vi "storage.vi"(8 "error in (no error)":errorcluster, 11 "reference in":refnum<class "Project Panels.lvclass">=refnum) -> (0 "error out":errorcluster={"status"=TRUE, "code"=1556, "source"="In Place Element Structure in Project Panels.lvclass:items.vi"}, 2 "saved?":bool, 3 "reference out":refnum<class "Project Panels.lvclass">)   [LabVIEW 2015, in "Project Panels.lvclass"]
uses:
  Project Panels.lvclass
  SYS/Items Controller_llb/storageSheets.ctl
  stateItem.ctl
  <vilib>/Utility/miscctls.llb/LVRowAndColumnUnsignedTypeDef.ctl
  <vilib>/Utility/miscctls.llb/LVRowAndColumnTypeDef.ctl
  SYS/Items Controller_llb/Items Controller.lvclass
  SYS/File Controller_llb/File Controller.lvclass
panel:
  out "title":string="Cosmed Asia Pacific - Storage"
  in  "tables":enum32{"Check IN", "Check OUT", "Storage"}(tab)
  in  "checkIN":string[][](table)
  in  "checkOUT":string[][](table)
  in  "Storage":string[][](table)
  in  "uploadFile":bool
  in  "Add Check OUT":bool
  in  "Add Check IN":bool
  out "Number of Items:":i32
  out "index":i32
  in  "back":bool
  in  "next":bool
  out "storageSheets":T1
  in  "Search Item":bool
  in  "Save":bool
  out "Item Selected (S/N or P/N):":string
  out "statuBar":string="Stoped for an Error"
  in  "Stop Button":bool
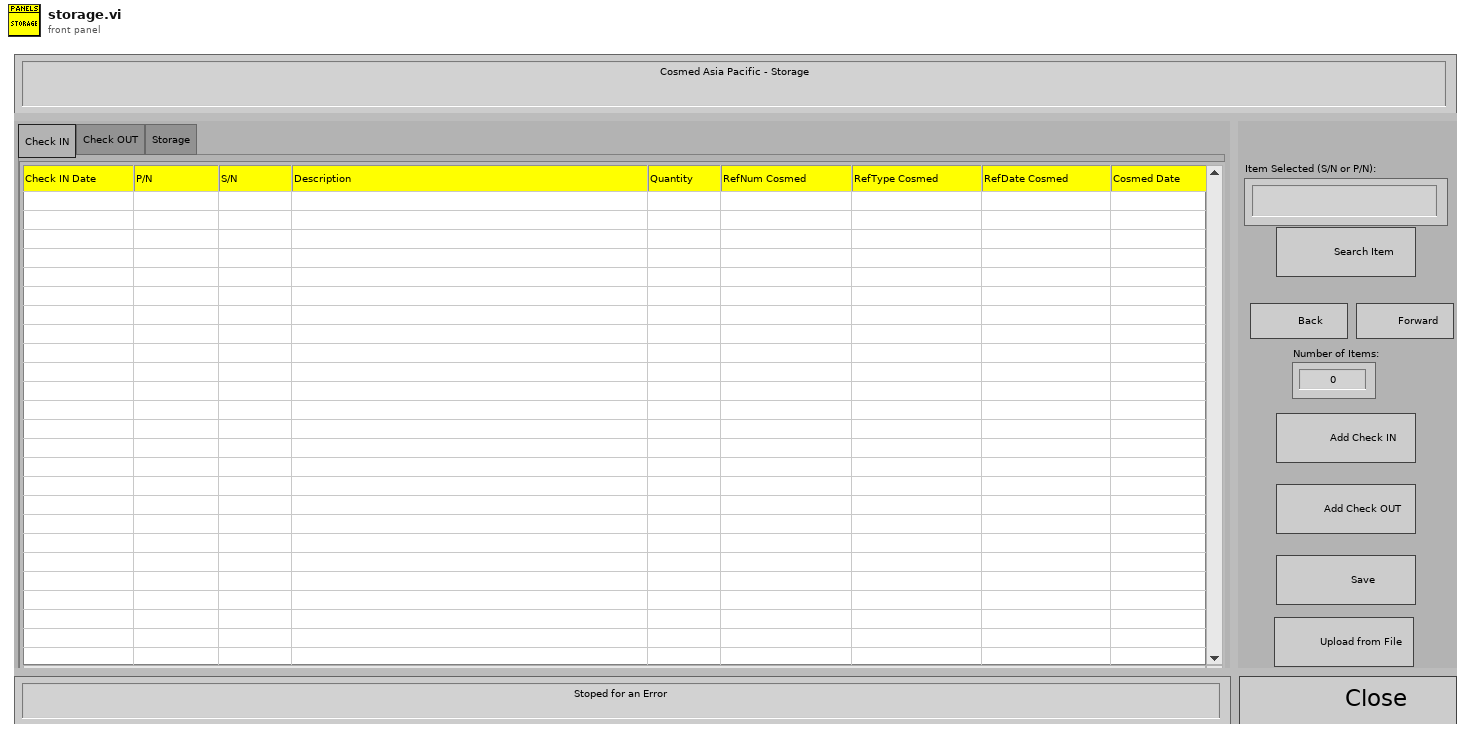
[diagram p1: front panel]
types:
  T1 = typedef "Items Controller.lvclass/storageSheets.ctl" = enum16{"check-in", "check-out", "storage"}
  T2 = typedef "Project Panels.lvclass/stateItem.ctl" = enum16{"initiate", "waitEvent", "save", "search", "UploadFile", "nextItems", "stop"}
  T3 = typedef "LVRowAndColumnUnsignedTypeDef.ctl" = cluster{"Row":u32, "Column":u32}
  T4 = enum8{"Enabled", "Disabled", "Disabled and Grayed Out"}
  T5 = cluster{"checkIN":string[][], "checkOUT":string[][], "storage":string[][]}
  T6 = typedef "LVRowAndColumnTypeDef.ctl" = cluster{"Row":i32, "Column":i32}
  T7 = typedef "Project Panels.lvclass/ObjectAttributesRef.ctl" = refnum<data-value>
  T8 = typedef "Project Panels.lvclass/ObjectAttributes.ctl" = cluster{"MyAttribute":dbl, "device_controller_ref":refnum<class "Devices Controller.lvclass">, "file_controller_ref":refnum<class "File Controller.lvclass">, "item_controller_ref":refnum<class "Items Controller.lvclass">, "item_tables":cluster{"checkIN":string[][], "checkOUT":string[][], "storage":string[][]}, "quickbook_table":cluster{"notes":string[][]}, "notification_controller_ref":refnum<class "Notification Controller.lvclass">, "partstracking_controller_ref":refnum<class "PartsTracking Controller.lvclass">, "product_tables":cluster{"k4b2":string[][], "fitmate":string[][], "RMR":string[][], "CPET":string[][], "BP":string[][], "PP":string[][], "k5":string[][], "bb-pft":string[][]}, "rowsColour":u32[], "low_resolution?":bool, "run_python?":bool}
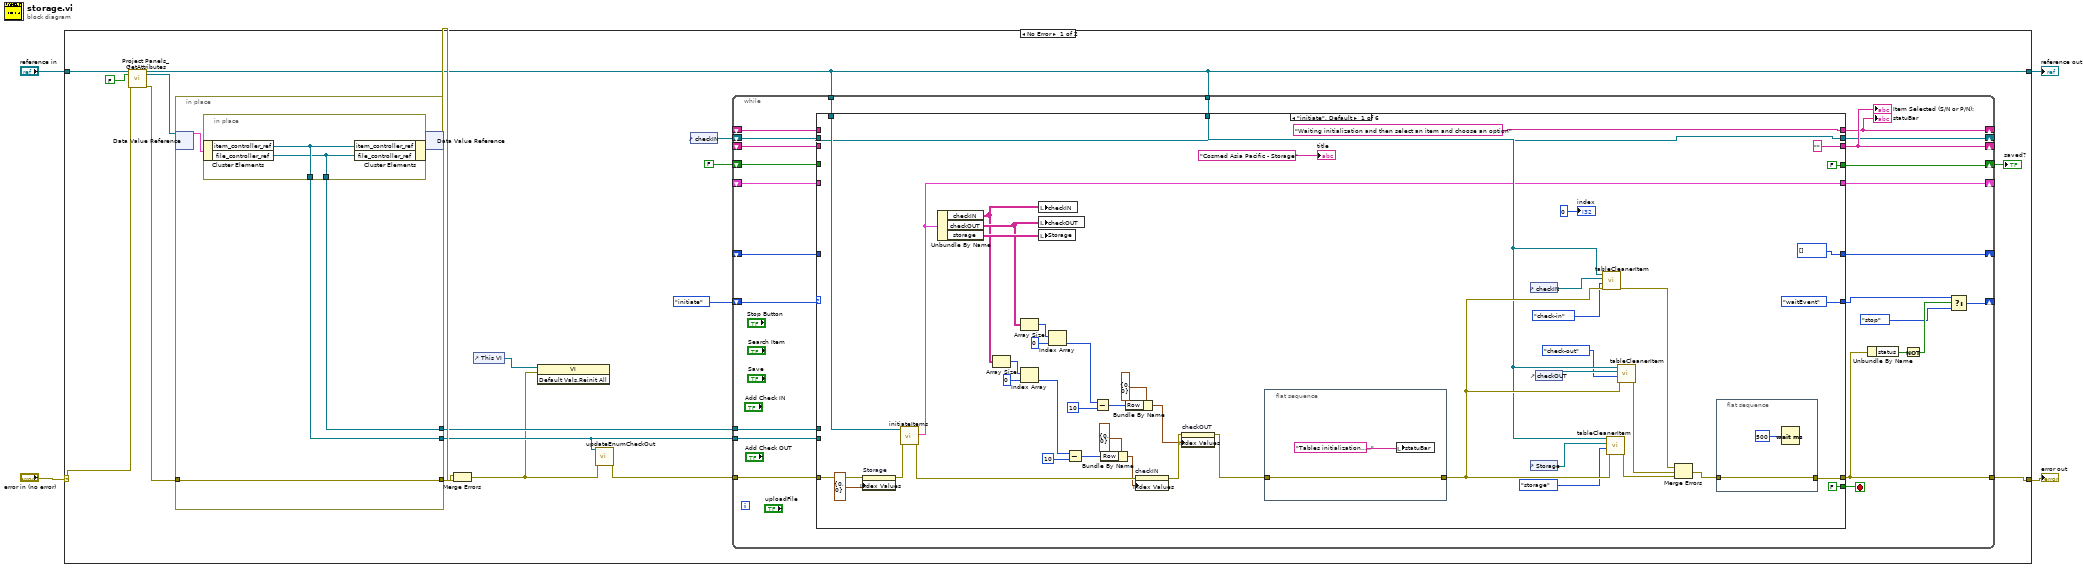
[diagram p0: block diagram]
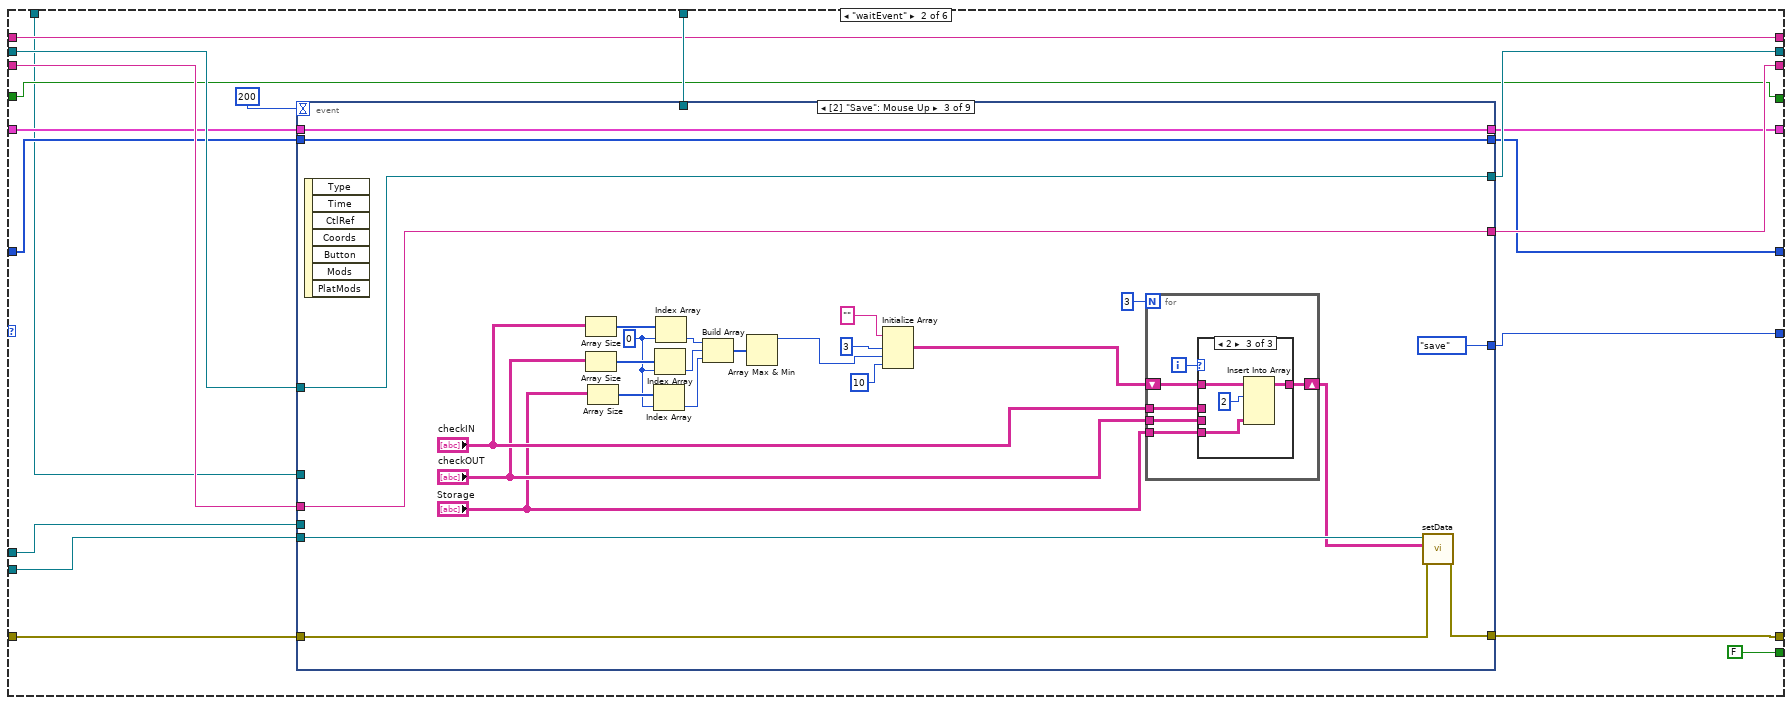
[diagram p2: hidden frame]
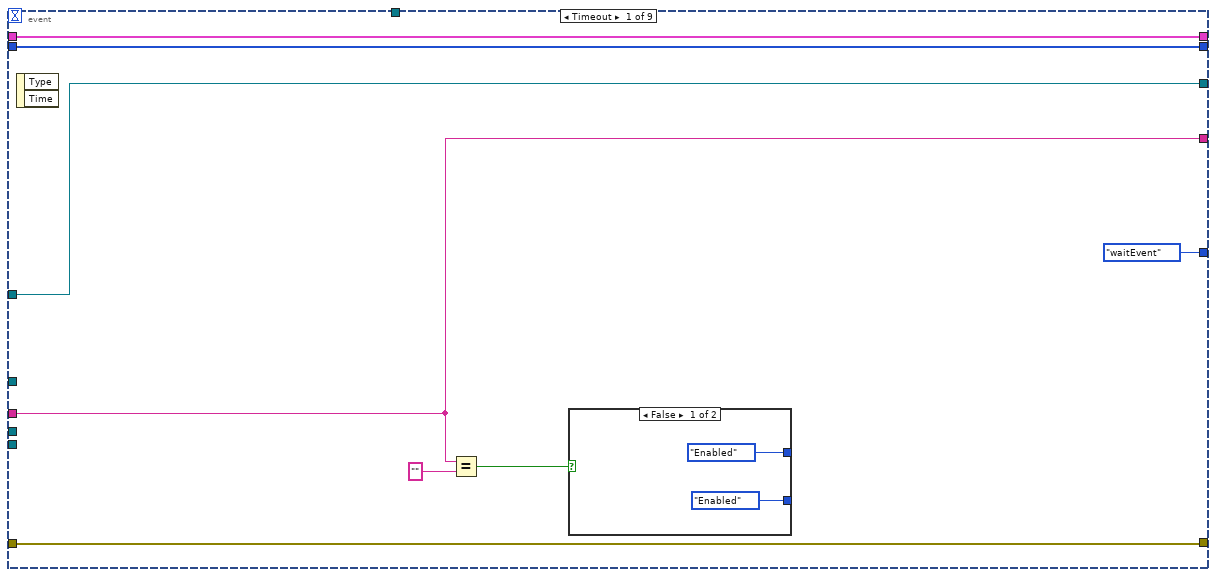
[diagram p3: hidden frame]
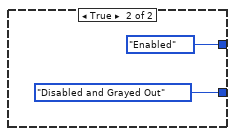
[diagram p4: hidden frame]
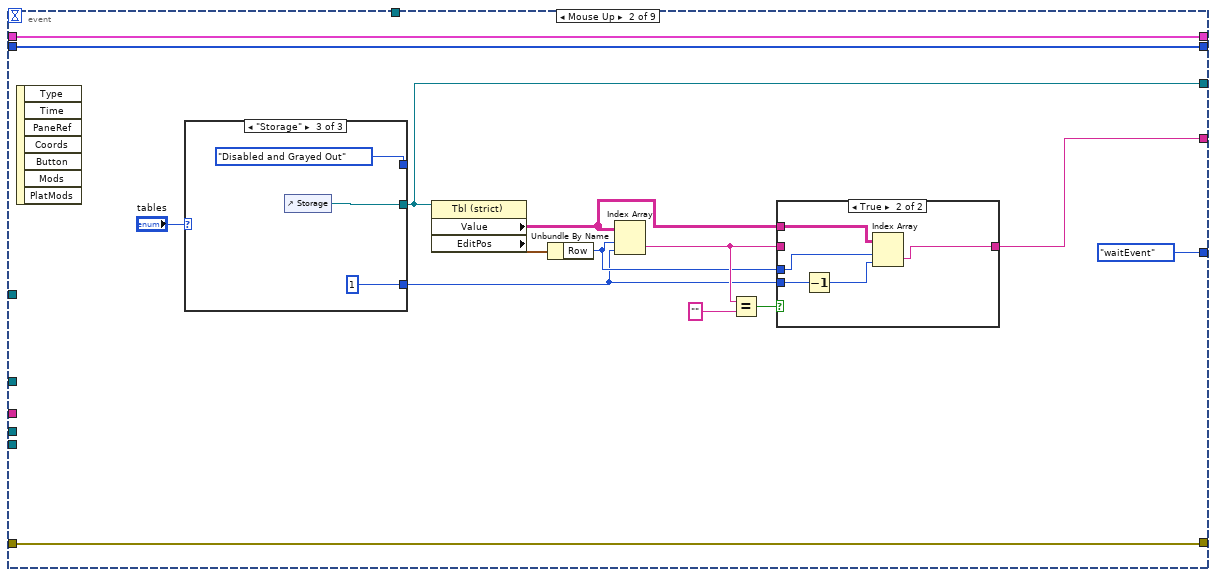
[diagram p5: hidden frame]
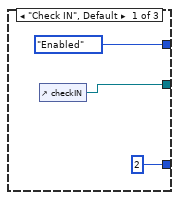
[diagram p7: hidden frame]
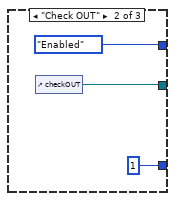
[diagram p8: hidden frame]
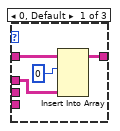
[diagram p9: hidden frame]
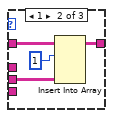
[diagram p10: hidden frame]
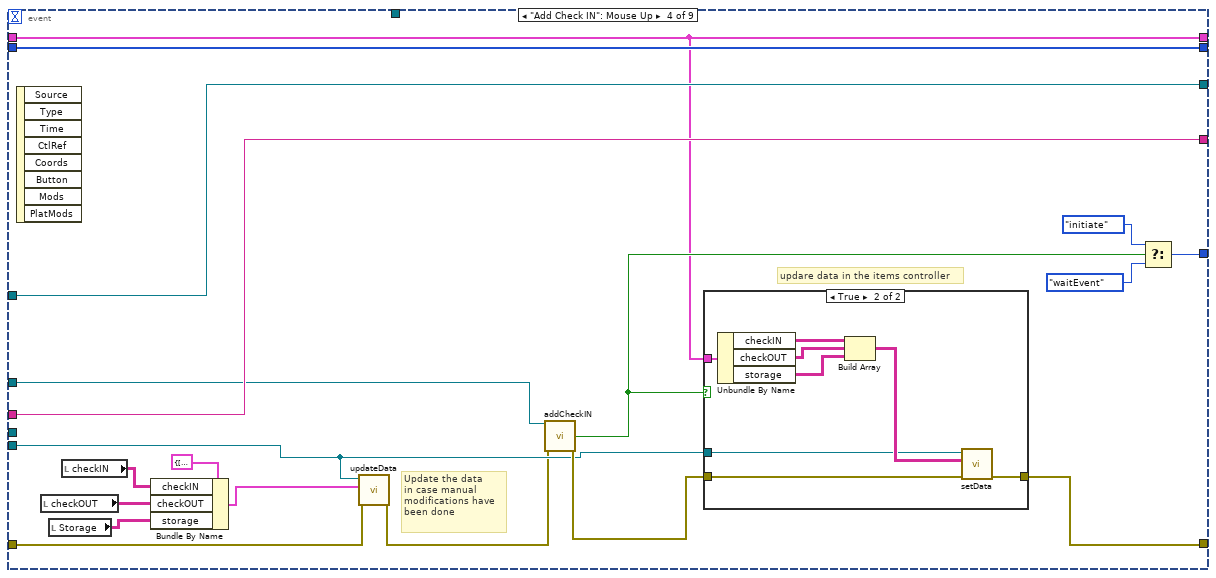
[diagram p11: hidden frame]
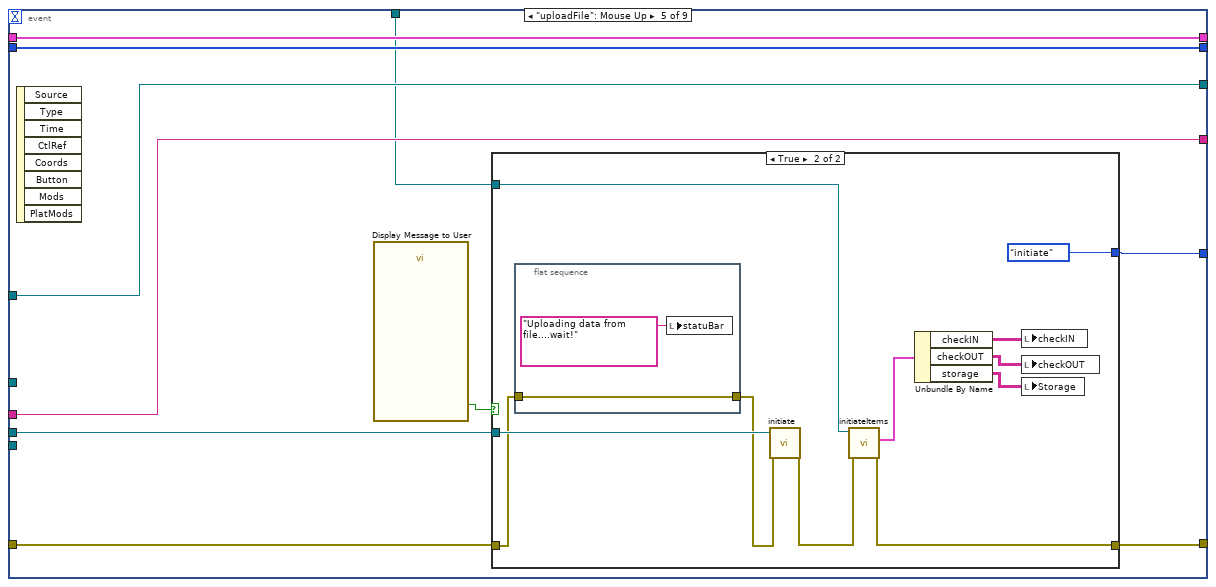
[diagram p13: hidden frame]
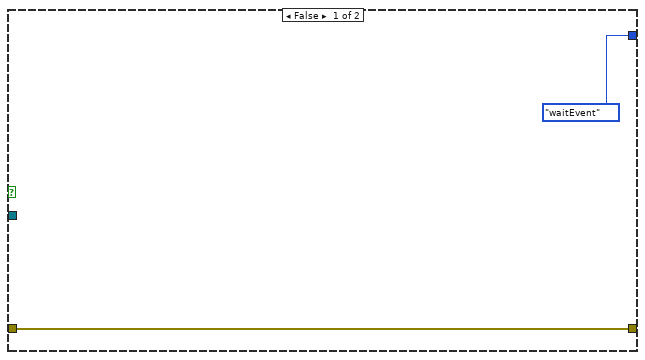
[diagram p14: hidden frame]
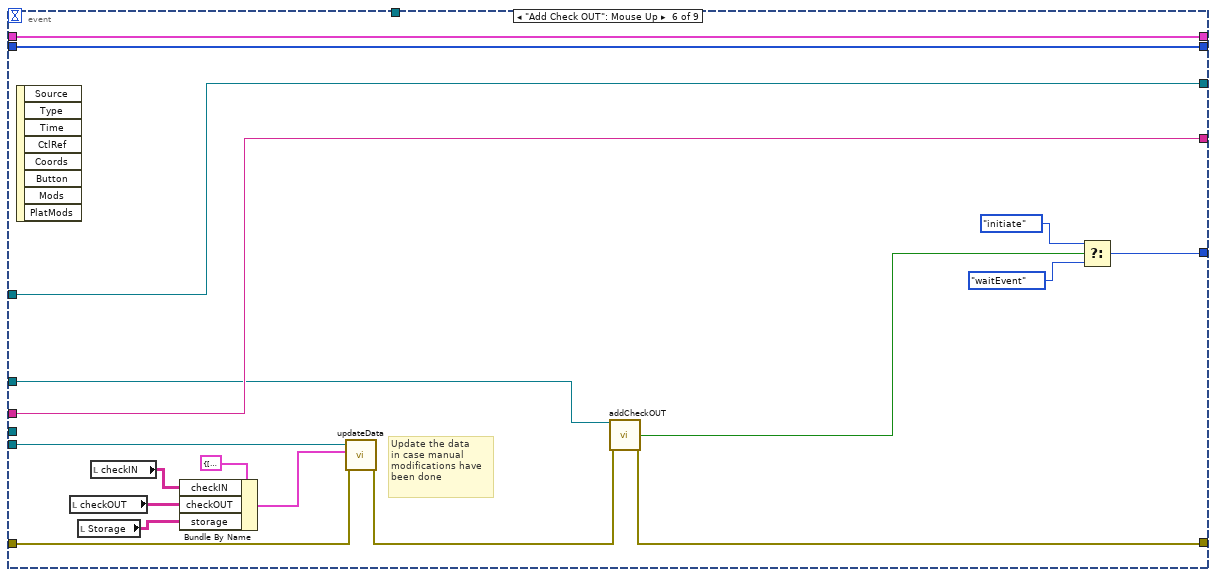
[diagram p15: hidden frame]
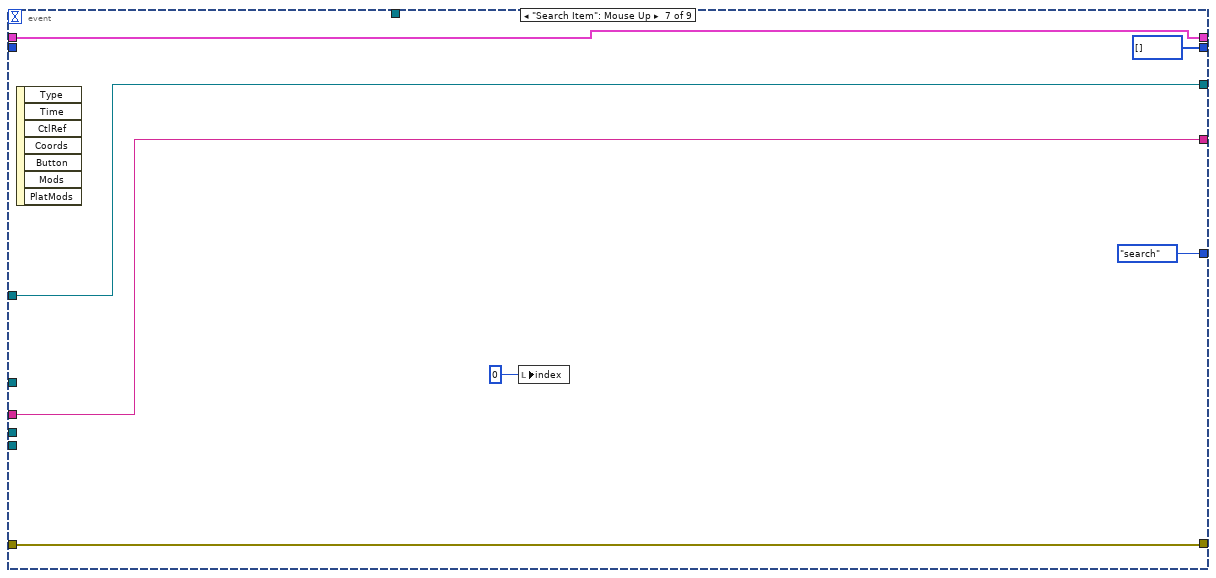
[diagram p16: hidden frame]
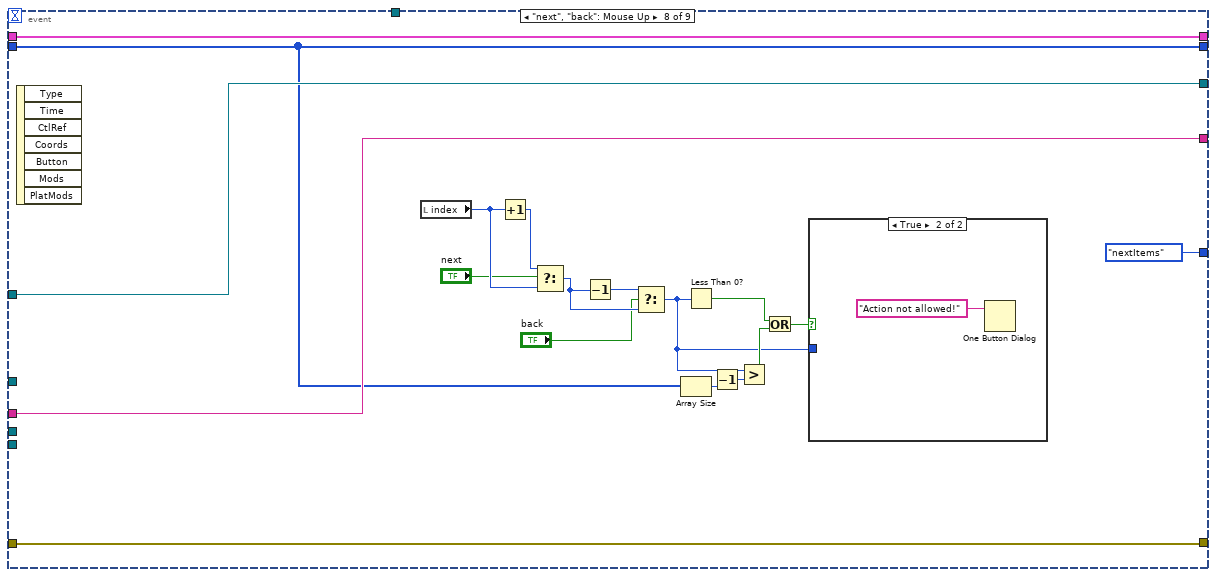
[diagram p17: hidden frame]
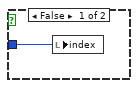
[diagram p18: hidden frame]
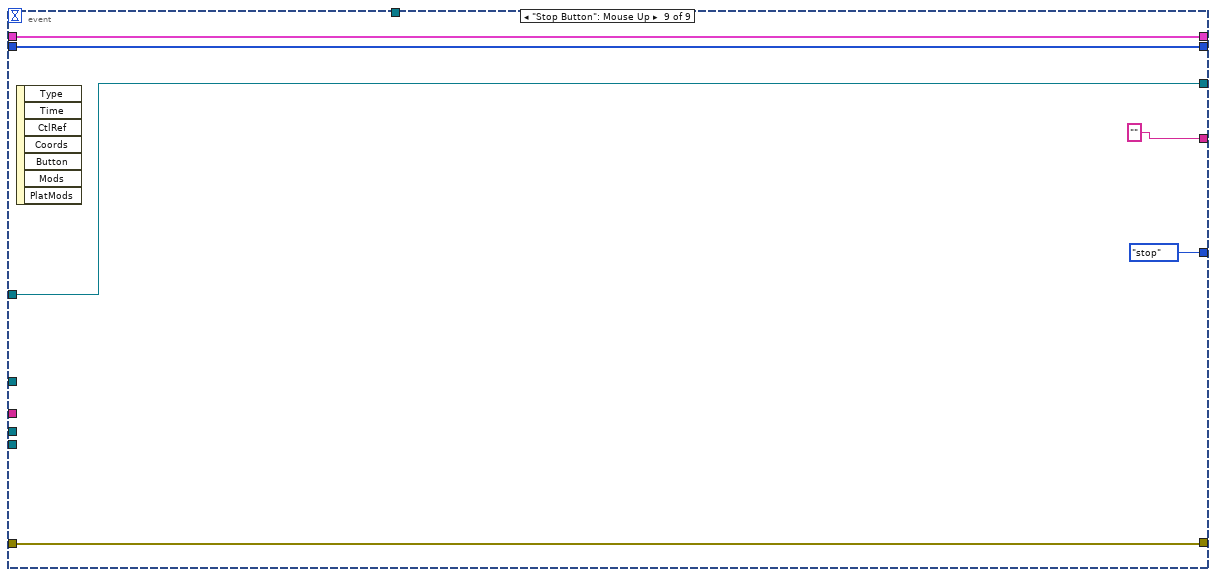
[diagram p19: hidden frame]
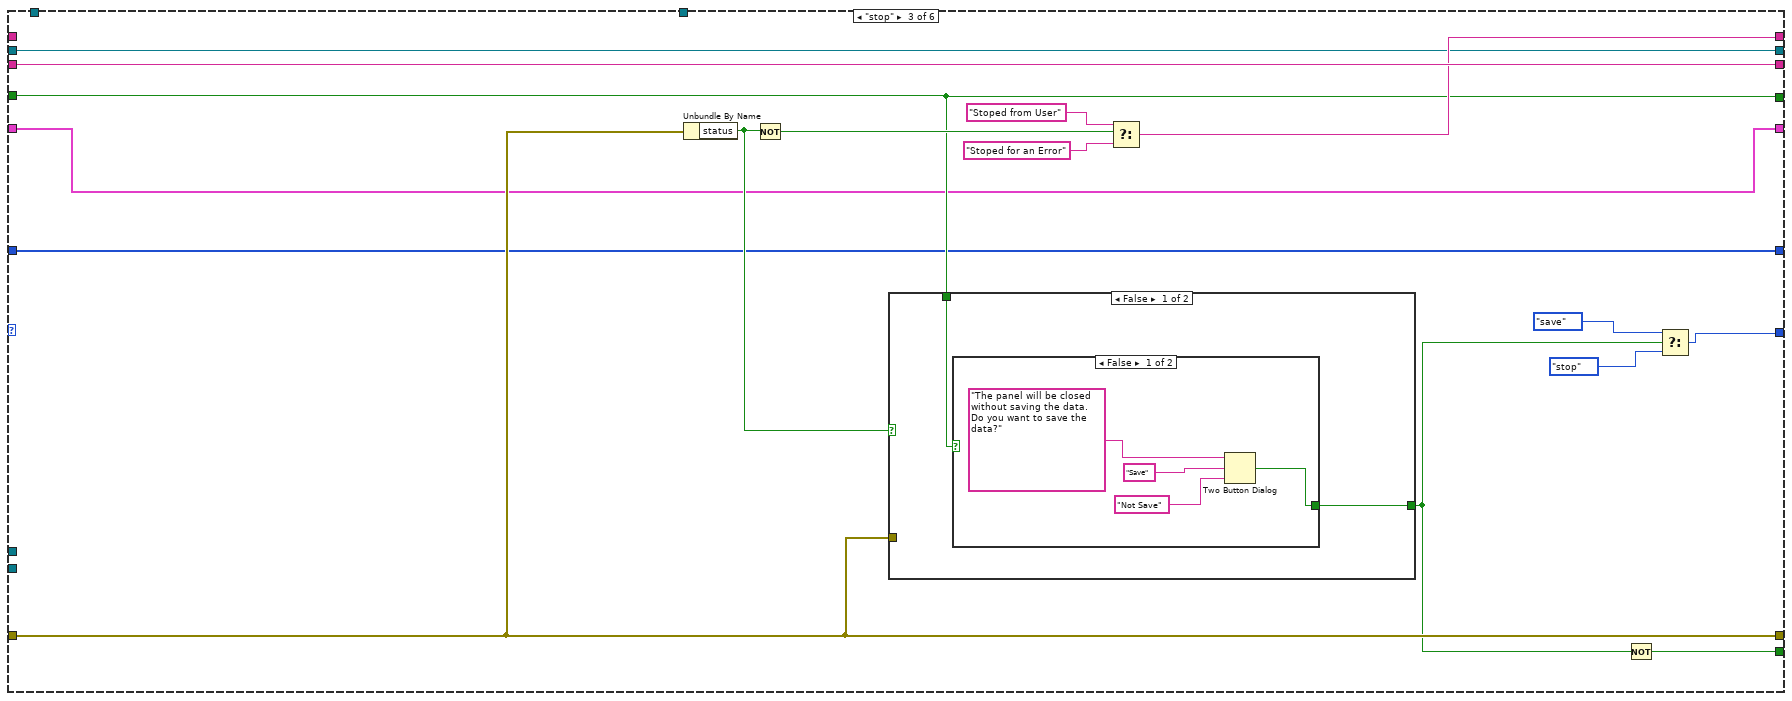
[diagram p20: hidden frame]
diagram:
  n1 = case shown="No Error" "error in (no error)" {
    selector: "error in (no error)" -> [w18 w401]
    tunnel: [w15 w401] -> w3
    tunnel: [w13 w400] -> w1
    tunnel: "reference in" -> [w20 w400]
    frame No Error {
      n2 = call "Project Panels_GetAttributes.vi"("reference in"=w20, "return data? (T)"=FALSE, "error in (no error)"=w18) -> ("reference out"=w13:refnum<class "Project Panels.lvclass">, "attributes ref"=w16:T7, "error out"=w17:errorcluster)  [unwired: 13 in, 1 out]
      n3 = in-place {
        in-place-border: w17 -> [w395]
        in-place-border: [w395] -> w21
        in-place-border: [w394] -> w7
        in-place-border: [w393] -> w8
        n4 = in-place-dvr #1(w16) -> (w396:T8)  [unwired: 1 out]
        n5 = in-place {
          in-place-border: [w399] -> w394
          in-place-border: [w398] -> w393
          n6 = in-place-cluster #2(w396) -> ("item_controller_ref"=w399:refnum<class "Items Controller.lvclass">, "file_controller_ref"=w398:refnum<class "File Controller.lvclass">)
          n7 = in-place-cluster #2("item_controller_ref"=w399, "file_controller_ref"=w398) -> (w397:T8)
        }
        n8 = in-place-dvr #1(w397) -> (w22:errorcluster)  [unwired: 1 out]
      }
      n9 = Merge Errors(w21, w22) -> (w6:errorcluster)
      n10 = control-ref of="This VI"() -> (w11:refnum<vi>)
      n11 = invoke class="VI" method="Default Vals.Reinit All"(reference=w11, error in=w6) -> ()  [unwired: 1 in, 3 out]
      n12 = call "updateEnumCheckOut.vi"("reference in"=w7, "error in (no error)"=w6) -> ("error out"=w5:errorcluster)  [unwired: 16 in, 1 out]
      n13 = control-ref of="checkIN"() -> (w12:refnum<vi>)
      n14 = while {
        tunnel: w13 -> [w47]
        tunnel: w5 -> [w46]
        tunnel: [w44] -> w15
        shift-right: [w41] -> _
        shift-left: stateItem."initiate" ("state") -> [w45]
        shift-right: [w38] -> _
        shift-left: _ -> [w37]
        shift-right: [w36] -> _
        shift-left: w12 -> [w35]
        tunnel: w13 -> [w34]
        tunnel: w7 -> [w32]
        shift-right: [w30] -> w9
        shift-left: FALSE -> [w31]
        shift-right: [w29] -> _
        shift-left: _ -> [w28]
        shift-right: [w27] -> _
        shift-left: _ -> [w26]
        shift-right: [w25] -> _
        shift-left: _ -> [w24]
        tunnel: w8 -> [w23]
        stop <- w39 stop-if-true
        n15 = case shown="\"initiate\", Default" w45 {
          tunnel: w47 -> [w82 w107 _ _ _ _]
          tunnel: w46 -> [w75 w116 w317 w335 w367 w383]
          tunnel: [w85 w110 w317 w346 w367 w379] -> w44
          tunnel: [stateItem."waitEvent" ("state") w109 w312 w341 stateItem."waitEvent" ("state") stateItem."waitEvent" ("state")] -> w42
          tunnel: [FALSE FALSE w310 FALSE FALSE FALSE] -> w39
          tunnel: ["Waiting initialization and then select an item and choose an option" ("title") w105 w319 "Search Item option selected..." ("title") "Click on the arrows to select other items" ("title") w378] -> w29
          tunnel: ["" w112 w322 w347 w364 w385] -> w38
          tunnel: w37 -> [_ w114 w322 w347 w364 w385]
          tunnel: [w79 w111 w318 w348 w358 w386] -> w36
          tunnel: w35 -> [w79 w113 w318 w348 w358 w386]
          tunnel: w34 -> [w81 w100 _ w337 _ _]
          tunnel: w32 -> [_ w108 _ _ _ w384]
          tunnel: w31 -> [_ w106 w309 w345 w365 _]
          tunnel: [FALSE w106 w309 w345 w365 TRUE] -> w30
          tunnel: w28 -> [_ w105 _ _ _ _]
          tunnel: [i32[] [] ("indexElements") w103 w308 w339 w359 w380] -> w27
          tunnel: w26 -> [_ w104 w308 _ w359 w380]
          tunnel: [w48 w101 w307 w336 w351 w377] -> w25
          tunnel: w24 -> [_ w102 w307 w336 w351 w377]
          tunnel: w23 -> [_ w99 _ _ _ _]
          frame "initiate", Default {
            n16 = property on="Storage" class="Tbl (strict)"(error in=w75, "Index Values"=T3 {"Row"=0, "Column"=0}) -> (error out=w74:errorcluster)  [unwired: 1 in, 1 out]
            n17 = call "initiateItems.vi"("error in (no error)"=w74, "reference in"=w81) -> ("error out"=w66:errorcluster, "table"=w48:T5)  [unwired: 7 in, 1 out]
            n18 = Unbundle By Name(w48) -> ("checkIN"=w49:string[][], "checkOUT"=w68:string[][], "storage"=w73:string[][])
            n19 = Array Size(array=w49) -> (size(s)=w55:i32[])
            n20 = Array Size(array=w68) -> (size(s)=w62:i32[])
            n21 = Index Array(array=w55, index=0) -> (element=w52:i32)
            n22 = local write "checkIN"(w49) -> ()
            n23 = local write "checkOUT"(w68) -> ()
            n24 = local write "Storage"(w73) -> ()
            n25 = Index Array(array=w62, index=0) -> (element=w59:i32)
            n26 = Subtract(x=w52, y=10) -> (x-y=w53:i32)
            n27 = Subtract(x=w59, y=10) -> (x-y=w60:i32)
            n28 = Bundle By Name(cluster=T3 {"Row"=0, "Column"=0} ("Index Values"), "Row"=w53) -> (w50:T3)
            n29 = Bundle By Name(cluster=T3 {"Row"=0, "Column"=0} ("Index Values"), "Row"=w60) -> (w57:T3)
            n30 = property on="checkIN" class="Tbl (strict)"(error in=w66, "Index Values"=w50) -> (error out=w65:errorcluster)  [unwired: 1 in, 1 out]
            n31 = property on="checkOUT" class="Tbl (strict)"(error in=w65, "Index Values"=w57) -> (error out=w67:errorcluster)  [unwired: 1 in, 1 out]
            n32 = flat-sequence {
              tunnel: w67 -> [w96]
              tunnel: [w96] -> w84
              frame #0 {
                n33 = local write "statuBar"("Tables initialization....." ("title")) -> ()
              }
            }
            n34 = control-ref of="checkIN"() -> (w92:refnum<vi>)
            n35 = control-ref of="Storage"() -> (w94:refnum<vi>)
            n36 = control-ref of="checkOUT"() -> (w93:refnum<vi>)
            n37 = call "tableCleanerItem.vi"("error in (no error)"=w84, "storageSheets"=storageSheets."check-in", "Table in"=w92, "reference in"=w82) -> ("error out"=w91:errorcluster)  [unwired: 6 in, 1 out]
            n38 = call "tableCleanerItem.vi"("error in (no error)"=w84, "storageSheets"=storageSheets."storage", "Table in"=w94, "reference in"=w82) -> ("error out"=w89:errorcluster)  [unwired: 6 in, 1 out]
            n39 = call "tableCleanerItem.vi"("error in (no error)"=w84, "storageSheets"=storageSheets."check-out", "Table in"=w93, "reference in"=w82) -> ("error out"=w90:errorcluster)  [unwired: 6 in, 1 out]
            n40 = Merge Errors(w91, w90, w89) -> (w80:errorcluster)
            n41 = flat-sequence {
              tunnel: w80 -> [w98]
              tunnel: [w98] -> w85
              frame #0 {
                n42 = Wait (ms)(milliseconds to wait=u32 500) -> ()  [unwired: 1 out]
              }
            }
            "title" <- "Cosmed Asia Pacific - Storage" ("title")
            "index" <- 0 ("index")
          }
          frame "waitEvent" {
            n43 = event shown="[2] \"Save\": Mouse Up" {
              selector: _ -> [_ _ _ _ _ _ _ _ _]
              dyn-events: _ -> [_ _ _ _ _ _ _ _ _]
              timeout: 200 -> [_ _ _ _ _ _ _ _ _]
              tunnel: w116 -> [w125 w143 w180 w209 w236 w264 w277 w298 w306]
              tunnel: [w125 w143 w179 w212 w235 w269 w277 w298 w306] -> w110
              tunnel: w114 -> [w121 _ w183 w221 w237 w273 w279 w291 _]
              tunnel: w113 -> [w122 _ w184 w220 w238 w272 w280 w292 w304]
              tunnel: [w121 w136 w183 w221 w237 w273 w279 w291 ""] -> w112
              tunnel: [w122 w140 w184 w220 w238 w272 w280 w292 w304] -> w111
              tunnel: [stateItem."waitEvent" ("state") stateItem."waitEvent" ("state") stateItem."save" ("state") w216 w233 w267 stateItem."search" ("state") stateItem."nextItems" ("state") stateItem."stop" ("state")] -> w109
              tunnel: w108 -> [_ _ w178 w211 _ w262 _ _ _]
              tunnel: w107 -> [_ _ _ _ w231 _ _ _ _]
              tunnel: w104 -> [w119 w131 w176 w219 w239 w271 _ w290 w302]
              tunnel: [w119 w131 w176 w219 w239 w271 i32[] [] ("indexElements") w290 w302] -> w103
              tunnel: w102 -> [w118 w130 w175 w210 w240 w261 w274 w281 w301]
              tunnel: [w118 w130 w175 w210 w240 w261 w274 w281 w301] -> w101
              tunnel: w100 -> [_ _ _ w218 _ w270 _ _ _]
              tunnel: w99 -> [_ _ _ _ w232 _ _ _ _]
              event Timeout {
                n44 = event-data() -> ()  [unwired: 1 in, 2 out]
                n45 = Equal?(x=w121, y="") -> (x = y?=w124:bool)
                n46 = case shown="False" w124 {
                  tunnel: [T4."Enabled" ("Disabled") T4."Disabled and Grayed Out" ("Disabled")] -> _
                  tunnel: [T4."Enabled" ("Disabled") T4."Enabled" ("Disabled")] -> _
                  frame False {
                  }
                  frame True {
                  }
                }
              }
              event Mouse Up {
                n47 = event-data() -> ()  [unwired: 1 in, 7 out]
                n48 = case shown="\"Storage\"" "tables" {
                  tunnel: [w152 w155 w158] -> w140
                  tunnel: [T4."Enabled" ("Disabled") T4."Enabled" ("Disabled") T4."Disabled and Grayed Out" ("Disabled")] -> _
                  tunnel: [2 ("disabled index (col)") 1 ("disabled index (col)") 1 ("disabled index (col)")] -> w133
                  frame "Check IN", Default {
                    n49 = control-ref of="checkIN"() -> (w152:refnum<vi>)
                  }
                  frame "Check OUT" {
                    n50 = control-ref of="checkOUT"() -> (w155:refnum<vi>)
                  }
                  frame "Storage" {
                    n51 = control-ref of="Storage"() -> (w158:refnum<vi>)
                  }
                }
                n52 = property on="Property Node" class="Tbl (strict)"(reference=w140) -> ("Value"=w135:string[][], "EditPos"=w142:T6)  [unwired: 1 in, 2 out]
                n53 = Unbundle By Name(w142) -> ("Row"=w134:i32)
                n54 = Index Array(array=w135, index (row)=w134, index (col)=w133) -> (element=w137:string)
                n55 = Equal?(x=w137, y="") -> (x = y?=w138:bool)
                n56 = case shown="True" w138 {
                  tunnel: w137 -> [w144 _]
                  tunnel: [w144 w145] -> w136
                  tunnel: w135 -> [_ w149]
                  tunnel: w134 -> [_ w148]
                  tunnel: w133 -> [_ w147]
                  frame False {
                  }
                  frame True {
                    n57 = Decrement(x=w147) -> (x-1=w146:i32)
                    n58 = Index Array(array=w149, index (row)=w148, index (col)=w146) -> (element=w145:string)
                  }
                }
              }
              event "Save": Mouse Up {
                w168 = 0 ("index")
                n59 = event-data() -> ()  [unwired: 1 in, 7 out]
                n60 = Array Size(array="checkIN") -> (size(s)=w171:i32[])
                n61 = Array Size(array="checkOUT") -> (size(s)=w170:i32[])
                n62 = Array Size(array="Storage") -> (size(s)=w169:i32[])
                n63 = Index Array(array=w169, index=w168) -> (element=w165:i32)
                n64 = Index Array(array=w170, index=w168) -> (element=w166:i32)
                n65 = Index Array(array=w171, index=w168) -> (element=w167:i32)
                n66 = Build Array(w167, w166, w165) -> (w164:i32[])
                n67 = Array Max & Min(array=w164) -> (max value=w161:i32)  [unwired: 3 out]
                n68 = Initialize Array("", 3 ("dimension size"), w161, 10 ("dimension size")) -> (w159:string[][][])
                n69 = for {
                  N: 3 -> [_]
                  shift-right: [w187] -> w177
                  shift-left: w159 -> [w189]
                  tunnel: "checkIN" -> [w188]
                  tunnel: "checkOUT" -> [w186]
                  tunnel: "Storage" -> [w185]
                  i -> [w190]
                  n70 = case shown="2" w190 {
                    tunnel: w189 -> [w194 w198 w202]
                    tunnel: w188 -> [w191 _ _]
                    tunnel: [w193 w197 w201] -> w187
                    tunnel: w186 -> [_ w195 _]
                    tunnel: w185 -> [_ _ w199]
                    frame 0, Default {
                      n71 = Insert Into Array(array=w194, index (dim 0)=0 ("index (page)"), new element=w191) -> (w193:string[][][])  [unwired: 2 in]
                    }
                    frame 1 {
                      n72 = Insert Into Array(array=w198, index (dim 0)=1 ("disabled index (page)"), new element=w195) -> (w197:string[][][])  [unwired: 2 in]
                    }
                    frame 2 {
                      n73 = Insert Into Array(array=w202, index (dim 0)=2 ("disabled index (page)"), new element=w199) -> (w201:string[][][])  [unwired: 2 in]
                    }
                  }
                }
                n74 = call "setData.vi"("error in (no error)"=w180, "data"=w177, "reference in"=w178) -> ("error out"=w179:errorcluster)  [unwired: 7 in, 1 out]
              }
              event "Add Check IN": Mouse Up {
                # "Update the data\nin case manual\nmodifications have\nbeen done"
                # "updare data in the items controller"
                n75 = event-data() -> ()  [unwired: 1 in, 8 out]
                n76 = local read "checkOUT"() -> (w205:string[][])
                n77 = local read "Storage"() -> (w204:string[][])
                n78 = local read "checkIN"() -> (w206:string[][])
                n79 = Bundle By Name(cluster=T5 {"checkIN"=[], "checkOUT"=[], "storage"=[]} ("table"), "checkIN"=w206, "checkOUT"=w205, "storage"=w204) -> (w203:T5)
                n80 = call "updateData.vi"("error in (no error)"=w209, "table"=w203, "reference in"=w211) -> ("error out"=w208:errorcluster)  [unwired: 7 in, 1 out]
                n81 = call "addCheckIN.vi"("reference in"=w218, "error in (no error)"=w208) -> ("saved?"=w214:bool, "error out"=w213:errorcluster)  [unwired: 11 in, 1 out]
                n82 = case shown="True" w214 {
                  tunnel: w210 -> [_ w226]
                  tunnel: w213 -> [w222 w225]
                  tunnel: [w222 w224] -> w212
                  tunnel: w211 -> [_ w223]
                  frame False {
                  }
                  frame True {
                    n83 = Unbundle By Name(w226) -> ("checkIN"=w230:string[][], "checkOUT"=w229:string[][], "storage"=w228:string[][])
                    n84 = Build Array(w230, w229, w228) -> (w227:string[][][])
                    n85 = call "setData.vi"("error in (no error)"=w225, "data"=w227, "reference in"=w223) -> ("error out"=w224:errorcluster)  [unwired: 7 in, 1 out]
                  }
                }
                n86 = Select(t=stateItem."initiate" ("state"), s=w214, f=stateItem."waitEvent") -> (s? t:f=w216:T2)
              }
              event "uploadFile": Mouse Up {
                n87 = event-data() -> ()  [unwired: 1 in, 8 out]
                n88 = call "Display Message to User"() -> ("Yes"=w234:bool)  [unwired: 10 in, 1 out]
                n89 = case shown="True" w234 {
                  tunnel: w236 -> [w242 w244]
                  tunnel: [w242 w248] -> w235
                  tunnel: [stateItem."waitEvent" ("state") stateItem."initiate" ("state")] -> w233
                  tunnel: w232 -> [_ w252]
                  tunnel: w231 -> [_ w250]
                  frame False {
                  }
                  frame True {
                    n90 = flat-sequence {
                      tunnel: w244 -> [w255]
                      tunnel: [w255] -> w243
                      frame #0 {
                        n91 = local write "statuBar"("Uploading data from file....wait!" ("statuBar")) -> ()
                      }
                    }
                    n92 = call "initiate.vi"("reference in"=w252, "error in (no error)"=w243) -> ("error out"=w249:errorcluster)  [unwired: 16 in, 1 out]
                    n93 = call "initiateItems.vi"("error in (no error)"=w249, "reference in"=w250) -> ("error out"=w248:errorcluster, "table"=w251:T5)  [unwired: 7 in, 1 out]
                    n94 = Unbundle By Name(w251) -> ("checkIN"=w247:string[][], "checkOUT"=w246:string[][], "storage"=w245:string[][])
                    n95 = local write "checkIN"(w247) -> ()
                    n96 = local write "checkOUT"(w246) -> ()
                    n97 = local write "Storage"(w245) -> ()
                  }
                }
              }
              event "Add Check OUT": Mouse Up {
                # "Update the data\nin case manual\nmodifications have\nbeen done"
                n98 = event-data() -> ()  [unwired: 1 in, 8 out]
                n99 = local read "checkOUT"() -> (w258:string[][])
                n100 = local read "Storage"() -> (w257:string[][])
                n101 = local read "checkIN"() -> (w259:string[][])
                n102 = Bundle By Name(cluster=T5 {"checkIN"=[], "checkOUT"=[], "storage"=[]} ("table"), "checkIN"=w259, "checkOUT"=w258, "storage"=w257) -> (w256:T5)
                n103 = call "updateData.vi"("error in (no error)"=w264, "table"=w256, "reference in"=w262) -> ("error out"=w263:errorcluster)  [unwired: 7 in, 1 out]
                n104 = call "addCheckOUT.vi"("reference in"=w270, "error in (no error)"=w263) -> ("saved?"=w266:bool, "error out"=w269:errorcluster)  [unwired: 11 in, 1 out]
                n105 = Select(t=stateItem."initiate" ("state"), s=w266, f=stateItem."waitEvent") -> (s? t:f=w267:T2)
              }
              event "Search Item": Mouse Up {
                n106 = event-data() -> ()  [unwired: 1 in, 7 out]
                n107 = local write "index"(0 ("index")) -> ()
              }
              event "next", "back": Mouse Up {
                n108 = event-data() -> ()  [unwired: 1 in, 7 out]
                n109 = local read "index"() -> (w296:i32)
                n110 = Increment(x=w296) -> (x+1=w297:i32)
                n111 = Select(t=w297, s="next", f=w296) -> (s? t:f=w294:i32)
                n112 = Decrement(x=w294) -> (x-1=w295:i32)
                n113 = Select(t=w295, s="back", f=w294) -> (s? t:f=w285:i32)
                n114 = Array Size(array=w290) -> (size(s)=w289:i32)
                n115 = Less Than 0?(x=w285) -> (x < 0?=w287:bool)
                n116 = Decrement(x=w289) -> (x-1=w282:i32)
                n117 = Greater?(x=w285, y=w282) -> (0:w288:bool)
                n118 = Or(x=w287, y=w288) -> (x .or. y?=w286:bool)
                n119 = case shown="True" w286 {
                  tunnel: w285 -> [w299 _]
                  frame False {
                    n120 = local write "index"(w299) -> ()
                  }
                  frame True {
                    n121 = One Button Dialog(message="Action not allowed!") -> ()  [unwired: 1 in, 1 out]
                  }
                }
              }
              event "Stop Button": Mouse Up {
                n122 = event-data() -> ()  [unwired: 1 in, 7 out]
              }
            }
          }
          frame "stop" {
            n123 = Unbundle By Name(w317) -> ("status"=w316:bool)
            n124 = Not(x=w316) -> (.not. x?=w315:bool)
            n125 = case shown="False" w316 {
              tunnel: w317 -> [_ w332]
              tunnel: [w324 FALSE ("Save")] -> w311
              tunnel: w309 -> [w323 _]
              frame False {
                n126 = case shown="False" w323 {
                  tunnel: [w327 FALSE ("Save")] -> w324
                  frame False {
                    n127 = Two Button Dialog(message="The panel will be closed without saving the data. Do you want to save the data?", 1:"Not Save" ("F button name (\"Cancel\")"), 2:"Save" ("T button name (\"OK\")")) -> (T button?=w327:bool)
                  }
                  frame True {
                  }
                }
              }
              frame True {
                n128 = Unbundle By Name(w332) -> ("source"=w331:string)
                n129 = Concatenate Strings("An Error occur: " ("message"), w331) -> (w334:string)
                n130 = One Button Dialog(message=w334) -> ()  [unwired: 1 in, 1 out]
              }
            }
            n131 = Select(t="Stoped from User" ("title"), s=w315, f="Stoped for an Error" ("title")) -> (s? t:f=w319:string)
            n132 = Not(x=w311) -> (.not. x?=w310:bool)
            n133 = Select(t=stateItem."save", s=w311, f=stateItem."stop" ("state")) -> (s? t:f=w312:T2)
          }
          frame "search" {
            n134 = call "searchItem.vi"("reference in"=w337, "error in (no error)"=w335) -> ("Sheet out"=→"storageSheets":T1, "indexElements"=w339:i32[], "error out"=w346:errorcluster)  [unwired: 10 in, 1 out]
            n135 = Array Size(array=w339) -> (size(s)=w338:i32)
            "Number of Items:" <- w338
            n136 = Greater Than 0?(x=w338) -> (x > 0?=w340:bool)
            n137 = Select(t=stateItem."nextItems" ("state"), s=w340, f=stateItem."waitEvent" ("state")) -> (s? t:f=w341:T2)
          }
          frame "nextItems" {
            n138 = local read "storageSheets"() -> (w354:T1)
            n139 = local read "index"() -> (w361:i32)
            n140 = case shown="\"storage\"" w354 {
              tunnel: [w369 w371 w373] -> w353
              tunnel: [enum32{"Check IN", "Check OUT", "Storage"}."Check IN" ("tables") enum32{"Check IN", "Check OUT", "Storage"}."Check OUT" ("tables") enum32{"Check IN", "Check OUT", "Storage"}."Storage" ("tables")] -> w352
              frame "check-in", Default {
                n141 = control-ref of="checkIN"() -> (w369:refnum<vi>)
              }
              frame "check-out" {
                n142 = control-ref of="checkOUT"() -> (w371:refnum<vi>)
              }
              frame "storage" {
                n143 = control-ref of="Storage"() -> (w373:refnum<vi>)
              }
            }
            n144 = Index Array(array=w359, index=w361) -> (element=w360:i32)
            n145 = Bundle By Name(cluster=T6 {"Row"=0, "Column"=0} ("Active Cell:Active Cell"), "Row"=w360, "Column"=0) -> (w355:T6)
            n146 = local write "tables"(w352) -> ()
            n147 = property on="Property Node" class="Tbl (strict)"(reference=w353, "Index Values"=w355) -> ()  [unwired: 1 in, 2 out]
          }
          frame "save" {
            n148 = flat-sequence {
              tunnel: w383 -> [w392]
              tunnel: [w392] -> w382
              frame #0 {
                n149 = local write "statuBar"("Saving...wait" ("title")) -> ()
              }
            }
            n150 = call "saveData.vi"("error in (no error)"=w382, "reference in"=w384) -> ("error out"=w375:errorcluster, "reference out"=w376:refnum<class "Items Controller.lvclass">)  [unwired: 8 in]
            n151 = call "updateEnumCheckOut.vi"("reference in"=w376, "error in (no error)"=w375) -> ("error out"=w374:errorcluster)  [unwired: 16 in, 1 out]
            n152 = flat-sequence {
              tunnel: w374 -> [w390]
              tunnel: [w390] -> w379
              tunnel: ["select an item and choose an option" ("title")] -> w378
              frame #0 {
              }
            }
          }
        }
        "statuBar" <- w29
        "Item Selected (S/N or P/N):" <- w38
        n153 = Unbundle By Name(w44) -> ("status"=w43:bool)
        n154 = Not(x=w43) -> (.not. x?=w40:bool)
        n155 = Select(t=w42, s=w40, f=stateItem."stop" ("state")) -> (s? t:f=w41:T2)
      }
      "saved?" <- w9
    }
    frame Error {
    }
  }
  "error out" <- w3
  "reference out" <- w1
